vi "obstacle_avoidance.vi"() -> ()   [LabVIEW 2017]
panel:
  in  "stop 2":bool
  out "distance in cm":dbl
  out "stop":bool
  out "move":bool
  in  "duration(micro seconds)":dbl
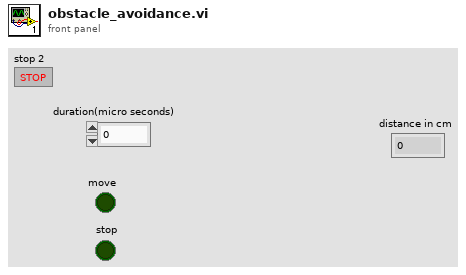
[diagram p1: front panel]
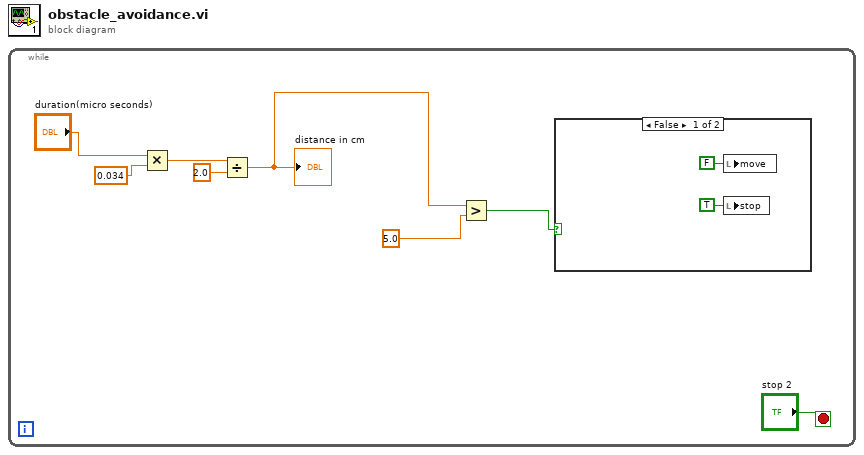
[diagram p0: block diagram]
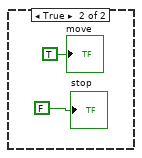
[diagram p2: hidden frame]
diagram:
  n1 = while {
    stop <- "stop 2" stop-if-true
    n2 = Multiply(x="duration(micro seconds)", y=0.034) -> (x*y=w5:dbl)
    n3 = Divide(x=w5, y=2.0) -> (x/y=w1:dbl)
    "distance in cm" <- w1
    n4 = Greater?(x=w1, y=5.0) -> (0:w2:bool)
    n5 = case shown="False" w2 {
      frame False {
        n6 = local write "move"(FALSE ("move")) -> ()
        n7 = local write "stop"(TRUE ("stop")) -> ()
      }
      frame True {
        "move" <- TRUE ("move")
        "stop" <- FALSE ("stop")
      }
    }
  }
